vi "ReadData.vi"(8 "Error In":errorcluster, 11 "reference in":refnum<class "FileDataSource.lvclass">) -> (0 "Error Out":errorcluster, 2 "Return(STRING)":string, 3 "reference out":refnum<class "FileDataSource.lvclass">)   [LabVIEW 2020, in "FileDataSource.lvclass"]
uses:
  FileDataSource.lvclass
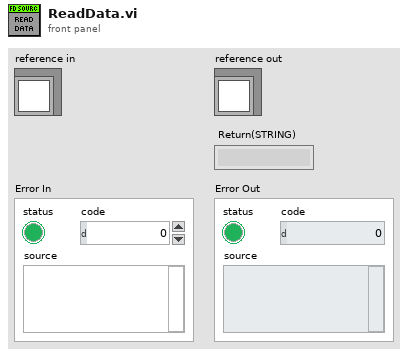
[diagram p1: front panel]
types:
  T1 = typedef "FileDataSource.lvclass/ObjectAttributes.ctl" = cluster{"Name":string}
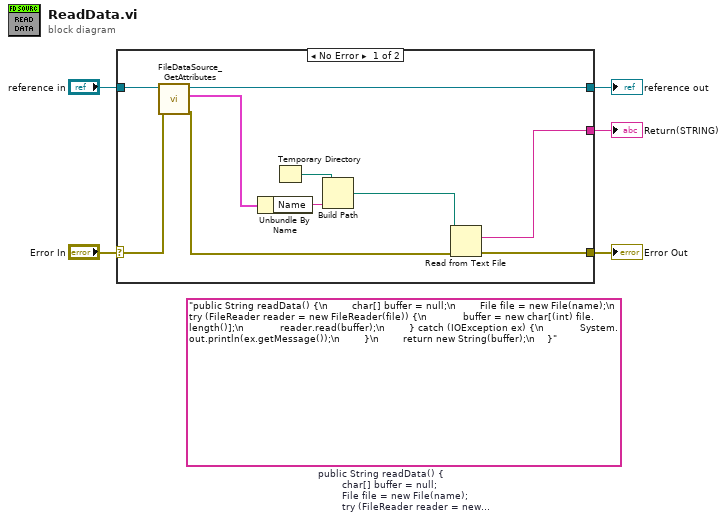
[diagram p0: block diagram]
diagram:
  (unwired) "public String readData() {\n        char[] buffer = null;\n        File file = new File(name);\n        try (FileReader reader = new FileReader(file)) {\n            buffer = new char[(int) file.length()];\n            reader.read(buffer);\n        } catch (IOException ex) {\n            System.out.println(ex.getMessage());\n        }\n        return new String(buffer);\n    }"  # public String readData() {         char[] buffer = null;         File file = new File(name);         try (FileReader reader = new FileReader(file)) {             buffer = new char[(int) file.length()];             reader.read(buffer);         } catch (IOException ex) {             System.out.println(ex.getMessage());         }         return new String(buffer);     }
  n1 = case shown="No Error" "Error In" {
    selector: "Error In" -> [w14 w17]
    tunnel: [w7 w17] -> w4
    tunnel: [w13 w16] -> w2
    tunnel: "reference in" -> [w15 w16]
    tunnel: [w6 _] -> w1
    frame No Error {
      n2 = call "FileDataSource_GetAttributes.vi"("error in (no error)"=w14, "reference in"=w15) -> ("error out"=w8:errorcluster, "Data"=w10:T1, "reference out"=w13:refnum<class "FileDataSource.lvclass">)  [unwired: 6 in, 1 out]
      n3 = Unbundle By Name(w10) -> ("Name"=w12:string)
      n4 = Temporary Directory() -> (w11:path)
      n5 = Build Path(base path=w11, name or relative path=w12) -> (appended path=w9:path)
      n6 = Read from Text File(file (use dialog)=w9, error in=w8) -> (text=w6:string, error out=w7:errorcluster)  [unwired: 2 in, 2 out]
    }
    frame Error {
    }
  }
  "Error Out" <- w4
  "reference out" <- w2
  "Return(STRING)" <- w1
